vi "Async Serial Engine.vi"(8 "error in (no error)":errorcluster, 10 "Engine Name":string, 11 "Varient Data":variant) -> (0 "error out":errorcluster)   [LabVIEW 2024]
doc: "All Rights Reserved © 2023 SyncSols"
uses:
  Controls/Async State Machine Cases.ctl
  Controls/Async Serial Configuration Cluster.ctl
  Main Engine/Controls/Main Engine JSON Command State.ctl
  Controls/Async Serial Command Q Cluster.ctl
  Main Engine/Controls/Main Engine Engine No.Options.ctl
  TCP Engine/Controls/TCP Engine Serial Interupt Cluster.ctl
  TCP Engine/TCP Engine.lvlib
  Controls/Async Message Info Cluster.ctl
  Controls/Async Frame Info Cluster.ctl
  Main Engine/Controls/Main Engine Q Option.ctl
  Controls/Async Sensor Type.ctl
  <vilib>/Modbus/master/Modbus Master.lvclass
  Controls/Async Serial State Machine Data Cluster.ctl
panel:
  in  "Data Cluster":T1={"Array"=[], "Boolean"=FALSE, "Varient Data"=variant(string ""), "Stop Notification"=refnum, "Start Notification"=refnum, "Command Q"=refnum, "Main Engine Response Q"=refnum, "TCP Engine Response Q"=refnum, "Engine Name"="", "Log File Refnum"=refnum, "Async serial Configuration Cluster"={"Port"="", "Minor Frame Freq"=0, "Minor Frame Count"=0, "Frame Info"=[], "Sensor Type"=0, "OIM Address"=0}, "VISA resource name"="", "Y"=[], "Rate"=0, "Dynamic Data?"=FALSE, "DyData Not Received"=FALSE, "Interupt Q"=refnum, "Modbus"=refnum} {"Async serial Configuration Cluster"."Minor Frame Count" min=5 max=8 step=1}
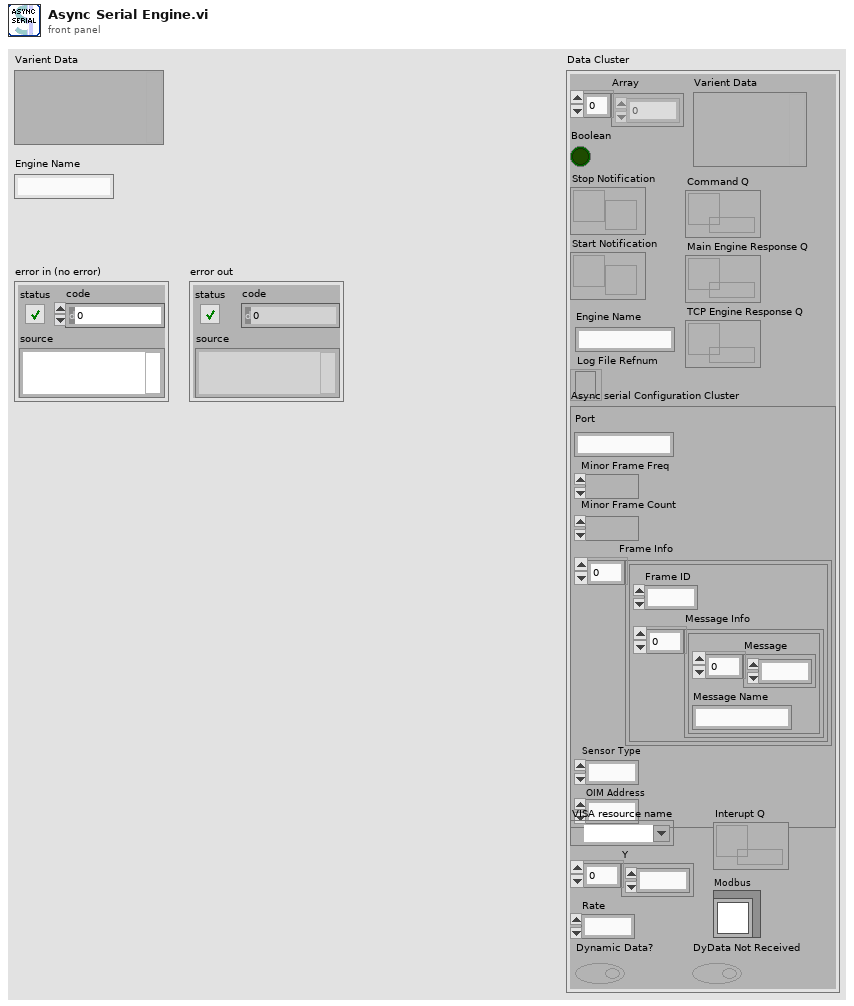
[diagram p1: front panel]
types:
  T1 = typedef "Async Serial State Machine Data Cluster.ctl" = cluster{"Array":dbl[], "Boolean":bool, "Varient Data":variant, "Stop Notification":refnum<notifier>, "Start Notification":refnum<notifier>, "Command Q":refnum<queue>, "Main Engine Response Q":refnum<queue>, "TCP Engine Response Q":refnum<queue>, "Engine Name":string, "Log File Refnum":refnum<file>, "Async serial Configuration Cluster":T2, "VISA resource name":refnum<visa-resource-name>, "Y":dbl[], "Rate":i32, "Dynamic Data?":bool, "DyData Not Received":bool, "Interupt Q":refnum<queue>, "Modbus":refnum<class "Modbus Master.lvclass">}
  T2 = typedef "Async Serial Configuration Cluster.ctl" = cluster{"Port":string, "Minor Frame Freq":u16, "Minor Frame Count":u16, "Frame Info":T3[], "Sensor Type":u16, "OIM Address":u16}
  T3 = typedef "Async Frame Info Cluster.ctl" = cluster{"Frame ID":u16, "Message Info":T4[]}
  T4 = typedef "Async Message Info Cluster.ctl" = cluster{"Message":u8[], "Message Name":string}
  T5 = typedef "Async State Machine Cases.ctl" = enum16{">Poll", ".........State Machine.........", ">Init", ">Error", ">Exit", "..........Async Serial..........", ">JSON to LVData", ">Gen Dyn Data", ">Configure", ">Get Command", ">Write Data"}
  T6 = typedef "Main Engine Q Option.ctl" = enum16{"Init", "Get"}
  T7 = typedef "TCP Engine.lvlib/TCP Engine Serial Interupt Cluster.ctl" = cluster{"Stop":bool, "JSON Variant":variant}
  T8 = typedef "Async Serial Command Q Cluster.ctl" = cluster{"Async serial Configuration Cluster":T2, "Command State":T9}
  T9 = typedef "Main Engine JSON Command State.ctl" = enum16{"Configure", "Start", "Exit"}
  T10 = typedef "Async Sensor Type.ctl" = enum16{"Camera", "INS", "Pri BMS", "Aux BMS", "Depth Sensor", "Altimeter", "OIM", "Thruster", "Acoustic Modem", "LED"}
  T11 = typedef "Main Engine Engine No.Options.ctl" = enum16{"Init", "Update", "Response", "Get"}
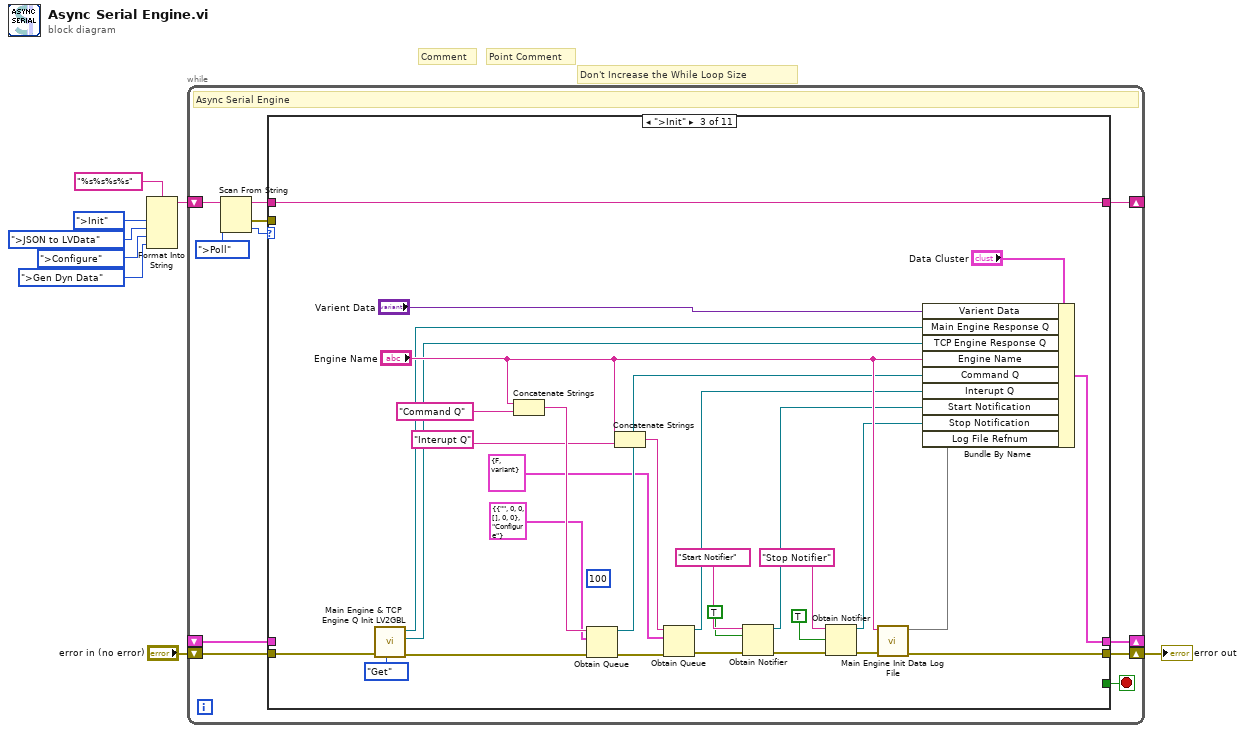
[diagram p0: block diagram]
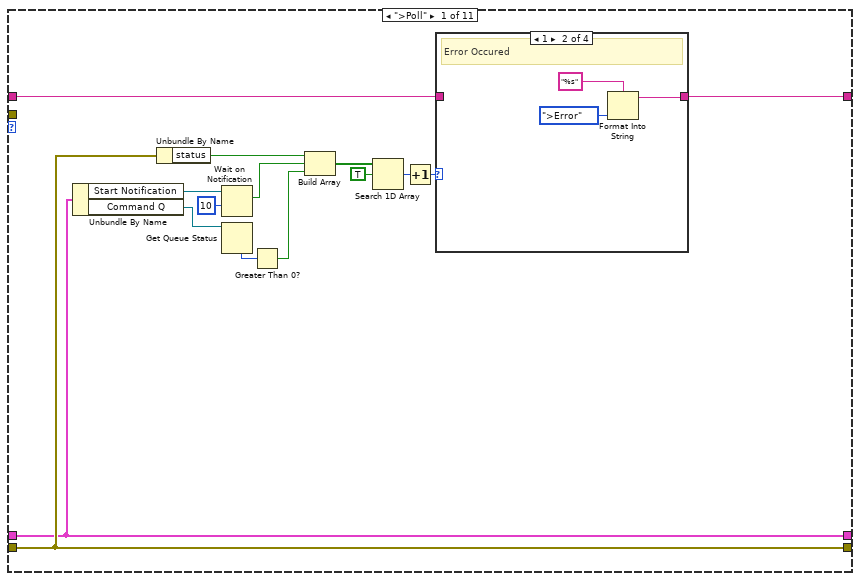
[diagram p2: hidden frame]
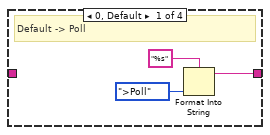
[diagram p3: hidden frame]
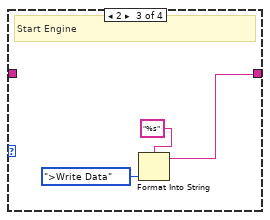
[diagram p4: hidden frame]
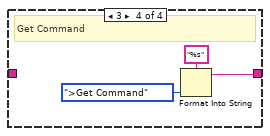
[diagram p5: hidden frame]
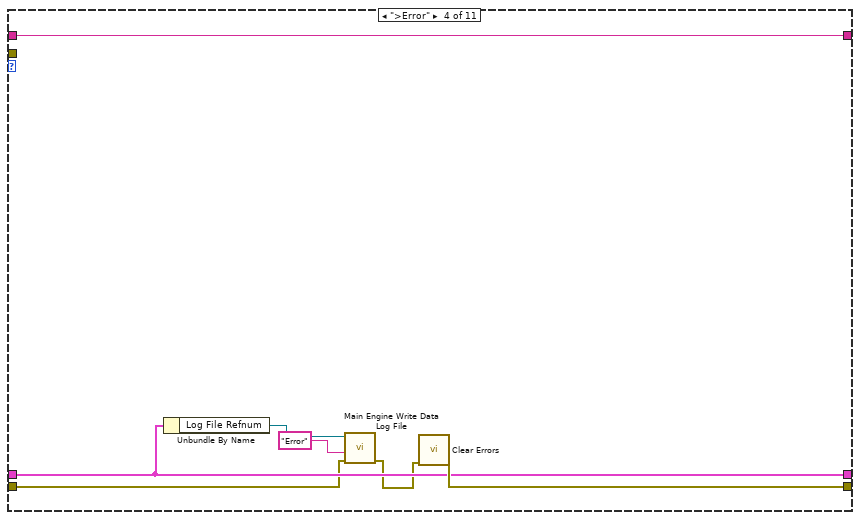
[diagram p7: hidden frame]
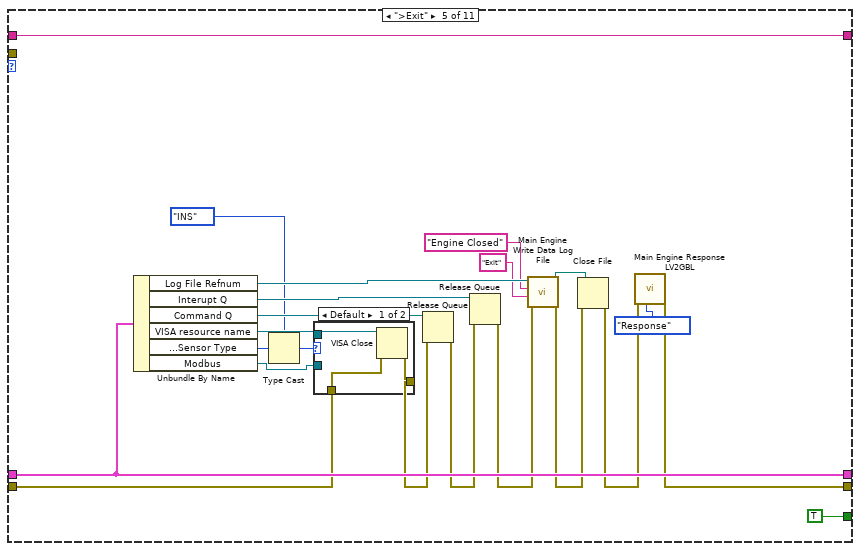
[diagram p8: hidden frame]
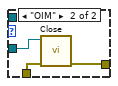
[diagram p9: hidden frame]
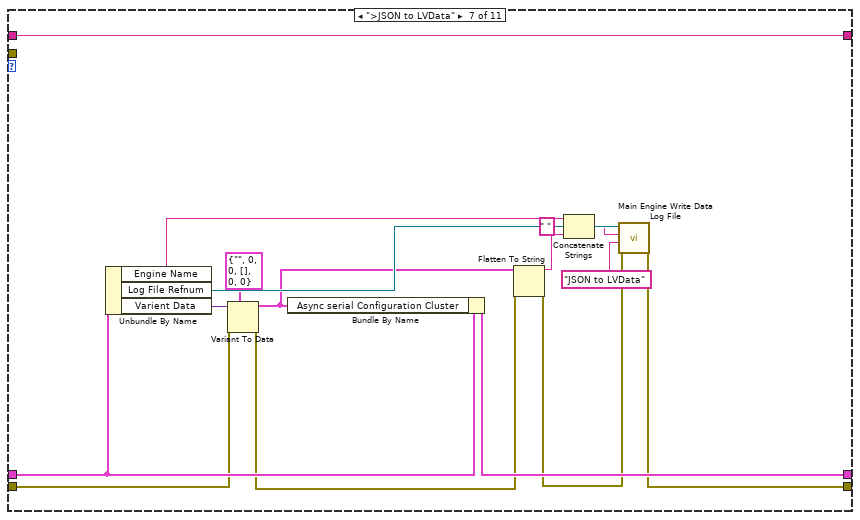
[diagram p11: hidden frame]
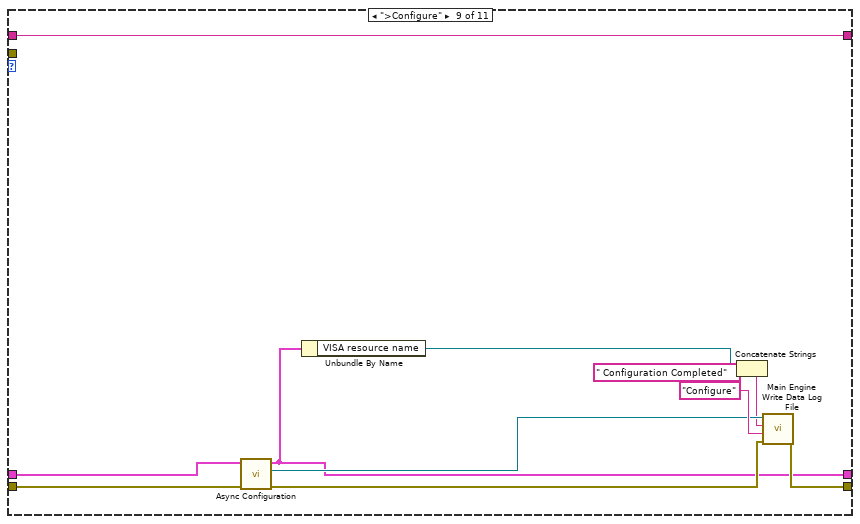
[diagram p13: hidden frame]
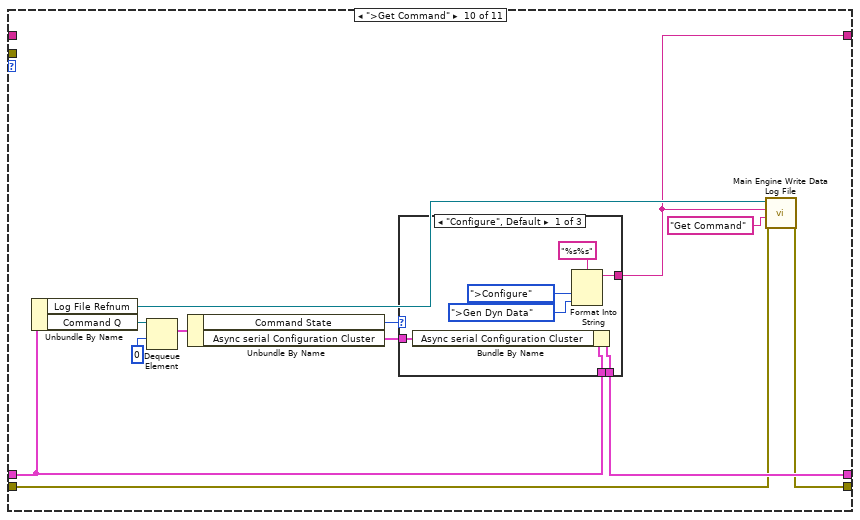
[diagram p14: hidden frame]
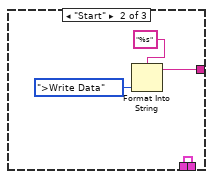
[diagram p15: hidden frame]
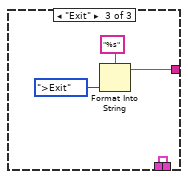
[diagram p16: hidden frame]
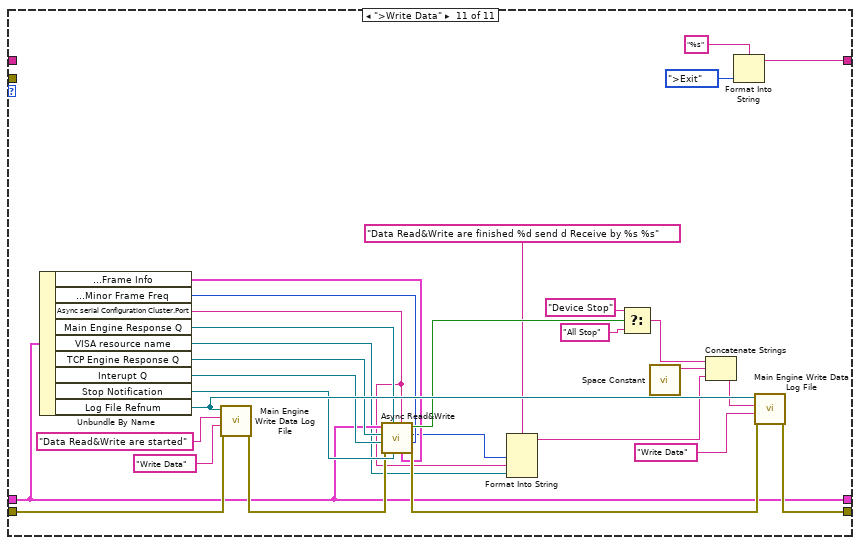
[diagram p17: hidden frame]
diagram:
  # "Don't Increase the While Loop Size"
  # "Point Comment"
  # "Comment"
  n1 = Format Into String(format string="%s%s%s%s", Async_State_Machine_Cases.">Init" ("SM Cases Options"), Async_State_Machine_Cases.">JSON to LVData" ("input 2"), Async_State_Machine_Cases.">Configure" ("input 3"), Async_State_Machine_Cases.">Gen Dyn Data" ("input 3")) -> (resulting string=w7:string)  [unwired: 2 in, 1 out]
  n2 = while {
    shift-right: [w14] -> _
    shift-left: w7 -> [w19]
    shift-right: [w12] -> w4
    shift-left: "error in (no error)" -> [w13]
    shift-right: [w10] -> _
    shift-left: _ -> [w9]
    stop <- w11 stop-if-true
    # "Async Serial Engine"
    n3 = Scan From String(input string=w19, default 1=Async_State_Machine_Cases.">Poll" ("SM Cases Options")) -> (remaining string=w15:string, error out=w17:errorcluster, output 1=w16:T5)  [unwired: 3 in, 1 out]
    n4 = case shown="\">Init\"" w16 {
      tunnel: w17 -> [_ _ _ _ _ _ _ _ _ _ _]
      tunnel: w15 -> [w34 w49 w79 w86 w108 w117 w133 w136 w142 _ _]
      tunnel: [w33 w49 w79 w86 w108 w117 w133 w136 w142 w151 w180] -> w14
      tunnel: w13 -> [w32 w48 w53 w81 w91 w116 w123 w135 w146 w148 w198]
      tunnel: [w32 w48 w65 w85 w95 w116 w128 w135 w144 w149 w203] -> w12
      tunnel: [_ _ _ _ TRUE _ _ _ _ _ _] -> w11
      tunnel: [w26 w47 w63 w82 w106 w115 w130 w134 w139 w154 w178] -> w10
      tunnel: w9 -> [w26 w47 _ w82 w106 w115 w132 w134 w147 w153 w178]
      frame ">Poll" {
        n5 = Unbundle By Name(w26) -> ("Start Notification"=w25:refnum<notifier>, "Command Q"=w24:refnum<queue>)
        n6 = Unbundle By Name(w32) -> ("status"=w31:bool)
        n7 = Wait on Notification(notifier=w25, timeout in ms (-1)=10) -> (notification=w23:bool)  [unwired: 2 in, 3 out]
        n8 = Get Queue Status(queue=w24) -> (# elements in queue=w21:i32)  [unwired: 2 in, 7 out]
        n9 = Greater Than 0?(x=w21) -> (x > 0?=w20:bool)
        n10 = Build Array(w31, w23, w20) -> (w30:bool[])
        n11 = Search 1D Array(1D array=w30, element=TRUE) -> (index of element=w28:i32)  [unwired: 1 in]
        n12 = Increment(x=w28) -> (x+1=w27:i32)
        n13 = case shown="1" w27 {
          tunnel: w34 -> [_ _ _ _]
          tunnel: [w35 w38 w43 w44] -> w33
          frame 0, Default {
            # "Default -> Poll"
            n14 = Format Into String(format string="%s", Async_State_Machine_Cases.">Poll" ("SM Cases Options")) -> (resulting string=w35:string)  [unwired: 2 in, 1 out]
          }
          frame 1 {
            # "Error Occured"
            n15 = Format Into String(format string="%s", Async_State_Machine_Cases.">Error" ("SM Cases Options")) -> (resulting string=w38:string)  [unwired: 2 in, 1 out]
          }
          frame 2 {
            # "Start Engine"
            n16 = Format Into String(format string="%s", Async_State_Machine_Cases.">Write Data" ("SM Cases Options")) -> (resulting string=w43:string)  [unwired: 2 in, 1 out]
          }
          frame 3 {
            # "Get Command"
            n17 = Format Into String(format string="%s", Async_State_Machine_Cases.">Get Command" ("SM Cases Options")) -> (resulting string=w44:string)  [unwired: 2 in, 1 out]
          }
        }
      }
      frame ".........State Machine........." {
      }
      frame ">Init" {
        (unwired) 100 ("max queue size (-1, unlimited)")
        n18 = call "Main Engine & TCP Engine Q Init LV2GBL.vi"("Q Option"=Main_Engine_Q_Option."Get", "error in"=w53) -> ("error out"=w54:errorcluster, "TCP Enigine Tx-Q"=w51:refnum<queue>, "Main Engine Tx-Q"=w52:refnum<queue>)  [unwired: 7 in]
        n19 = Concatenate Strings("Engine Name", "Command Q" ("name (unnamed)")) -> (w69:string)
        n20 = Obtain Queue(name (unnamed)=w69, element data type=T8 {"Async serial Configuration Cluster"={"Port"="", "Minor Frame Freq"=0, "Minor Frame Count"=0, "Frame Info"=[], "Sensor Type"=0, "OIM Address"=0}, "Command State"=enum."Configure"} ("Async Serial Command Q Cluster"), error in (no error)=w54) -> (queue out=w60:refnum<queue>, error out=w77:errorcluster)  [unwired: 2 in, 1 out]
        n21 = Concatenate Strings("Engine Name", "Interupt Q" ("name (unnamed)")) -> (w67:string)
        n22 = Obtain Queue(name (unnamed)=w67, element data type=T7 {"Stop"=FALSE, "JSON Variant"=variant} ("Serial Interupt Cluster"), error in (no error)=w77) -> (queue out=w55:refnum<queue>, error out=w76:errorcluster)  [unwired: 2 in, 1 out]
        n23 = Obtain Notifier(name (unnamed)="Start Notifier", notification data type=TRUE, error in (no error)=w76) -> (notifier out=w59:refnum<notifier>, error out=w75:errorcluster)  [unwired: 1 in, 1 out]
        n24 = Obtain Notifier(name (unnamed)="Stop Notifier", notification data type=TRUE, error in (no error)=w75) -> (notifier out=w58:refnum<notifier>, error out=w66:errorcluster)  [unwired: 1 in, 1 out]
        n25 = call "Main Engine Init Data Log File.vi"("error in"=w66, "Engine Name"="Engine Name") -> ("error out"=w65:errorcluster, 3:w57)  [unwired: 7 in, 1 out]
        n26 = Bundle By Name(cluster="Data Cluster", "Varient Data"="Varient Data", "Main Engine Response Q"=w52, "TCP Engine Response Q"=w51, "Engine Name"="Engine Name", "Command Q"=w60, "Interupt Q"=w55, "Start Notification"=w59, "Stop Notification"=w58, "Log File Refnum"=w57) -> (w63:T1)
      }
      frame ">Error" {
        n27 = Unbundle By Name(w82) -> ("Log File Refnum"=w84:refnum<file>)
        n28 = call "Main Engine Write Data Log File.vi"("error in"=w81, "State"="Error" ("Input Data"), "Log file path In"=w84) -> ("error out"=w80:errorcluster)  [unwired: 7 in, 1 out]
        n29 = call <vilib>:"Clear Errors.vi"("error in (no error)"=w80) -> ("error out"=w85:errorcluster)  [unwired: 5 in, 1 out]
      }
      frame ">Exit" {
        n30 = Unbundle By Name(w106) -> ("Log File Refnum"=w102:refnum<file>, "Interupt Q"=w93:refnum<queue>, "Command Q"=w103:refnum<queue>, "VISA resource name"=w92:refnum<visa-resource-name>, "Async serial Configuration Cluster.Sensor Type"=w90:u16, "Modbus"=w87:refnum<class "Modbus Master.lvclass">)
        n31 = Type Cast(type=Async_Sensor_Type."INS" ("Sensor Type"), x=w90) -> (*(type *) &x=w89:T10)
        n32 = case shown="Default" w89 {
          tunnel: [w111 w113] -> w105
          tunnel: w92 -> [w110 _]
          tunnel: w91 -> [w109 w114]
          tunnel: w87 -> [_ w112]
          frame Default {
            n33 = VISA Close(VISA resource name=w110, error in (no error)=w109) -> (error out=w111:errorcluster)
          }
          frame "OIM" {
            n34 = call-dynamic "Close.vi"("error in (no error)"=w114, "Modbus master in"=w112) -> ("error out"=w113:errorcluster)  [unwired: 9 in]
          }
        }
        n35 = Release Queue(queue=w103, error in (no error)=w105) -> (error out=w104:errorcluster)  [unwired: 1 in, 2 out]
        n36 = Release Queue(queue=w93, error in (no error)=w104) -> (error out=w101:errorcluster)  [unwired: 1 in, 2 out]
        n37 = call "Main Engine Write Data Log File.vi"("error in"=w101, "State"="Exit", "Input Data"="Engine Closed", "Log file path In"=w102) -> ("error out"=w100:errorcluster, "Log File Path Out"=w99:path)  [unwired: 6 in]
        n38 = Close File(refnum=w99, error in=w100) -> (error out=w96:errorcluster)  [unwired: 1 out]
        n39 = call "Main Engine Response LV2GBL.vi"("Options"=Main_Engine_Engine_No.Options."Response", "error in"=w96) -> ("error out"=w95:errorcluster)  [unwired: 7 in, 2 out]
      }
      frame "..........Async Serial.........." {
      }
      frame ">JSON to LVData" {
        n40 = Unbundle By Name(w132) -> ("Engine Name"=w119:string, "Log File Refnum"=w129:refnum<file>, "Varient Data"=w131:variant)
        n41 = Variant To Data(error in=w123, type=T2 {"Port"="", "Minor Frame Freq"=0, "Minor Frame Count"=0, "Frame Info"=[], "Sensor Type"=0, "OIM Address"=0} ("Async serial Configuration Cluster"), Variant=w131) -> (data=w121:T2, error out=w122:errorcluster)
        n42 = Bundle By Name(cluster=w132, "Async serial Configuration Cluster"=w121) -> (w130:T1)
        n43 = Flatten To String(anything=w121, error in (no error)=w122) -> (data string=w125:string, error out=w126:errorcluster)  [unwired: 2 in, 1 out]
        n44 = Concatenate Strings(w119, " " ("string"), w125) -> (w120:string)
        n45 = call "Main Engine Write Data Log File.vi"("error in"=w126, "State"="JSON to LVData", "Input Data"=w120, "Log file path In"=w129) -> ("error out"=w128:errorcluster)  [unwired: 6 in, 1 out]
      }
      frame ">Gen Dyn Data" {
      }
      frame ">Configure" {
        n46 = call "Async Configuration.vi"("error in"=w146, "Data Cluster in"=w147) -> ("error out"=w143:errorcluster, "File out"=w140:refnum<file>, "Data Cluster out"=w139:T1)  [unwired: 7 in]
        n47 = Unbundle By Name(w139) -> ("VISA resource name"=w137:refnum<visa-resource-name>)
        n48 = Concatenate Strings(w137, " Configuration Completed" ("Input Data")) -> (w138:string)
        n49 = call "Main Engine Write Data Log File.vi"("error in"=w143, "State"="Configure", "Input Data"=w138, "Log file path In"=w140) -> ("error out"=w144:errorcluster)  [unwired: 6 in, 1 out]
      }
      frame ">Get Command" {
        n50 = Unbundle By Name(w153) -> ("Log File Refnum"=w152:refnum<file>, "Command Q"=w159:refnum<queue>)
        n51 = Dequeue Element(queue=w159, timeout in ms (-1)=0) -> (element=w157:T8)  [unwired: 1 in, 3 out]
        n52 = Unbundle By Name(w157) -> ("Command State"=w156:T9, "Async serial Configuration Cluster"=w155:T2)
        n53 = case shown="\"Configure\", Default" w156 {
          tunnel: w153 -> [w166 w170 w174]
          tunnel: w155 -> [w165 _ _]
          tunnel: [w164 w170 w174] -> w154
          tunnel: [w161 w169 w171] -> w151
          frame "Configure", Default {
            n54 = Bundle By Name(cluster=w166, "Async serial Configuration Cluster"=w165) -> (w164:T1)
            n55 = Format Into String(format string="%s%s", Async_State_Machine_Cases.">Configure" ("SM Cases Options"), Async_State_Machine_Cases.">Gen Dyn Data" ("SM Cases Options")) -> (resulting string=w161:string)  [unwired: 2 in, 1 out]
          }
          frame "Start" {
            n56 = Format Into String(format string="%s", Async_State_Machine_Cases.">Write Data" ("SM Cases Options")) -> (resulting string=w169:string)  [unwired: 2 in, 1 out]
          }
          frame "Exit" {
            n57 = Format Into String(format string="%s", Async_State_Machine_Cases.">Exit" ("SM Cases Options")) -> (resulting string=w171:string)  [unwired: 2 in, 1 out]
          }
        }
        n58 = call "Main Engine Write Data Log File.vi"("error in"=w148, "State"="Get Command", "Input Data"=w151, "Log file path In"=w152) -> ("error out"=w149:errorcluster)  [unwired: 6 in, 1 out]
      }
      frame ">Write Data" {
        n59 = Unbundle By Name(w178) -> ("Async serial Configuration Cluster.Frame Info"=w184:T3[], "Async serial Configuration Cluster.Minor Frame Freq"=w183:u16, "Async serial Configuration Cluster.Port"=w176:string, "Main Engine Response Q"=w192:refnum<queue>, "VISA resource name"=w175:refnum<visa-resource-name>, "TCP Engine Response Q"=w191:refnum<queue>, "Interupt Q"=w190:refnum<queue>, "Stop Notification"=w189:refnum<notifier>, "Log File Refnum"=w199:refnum<file>)
        n60 = call "Main Engine Write Data Log File.vi"("error in"=w198, "State"="Write Data", "Input Data"="Data Read&Write are started", "Log file path In"=w199) -> ("error out"=w179:errorcluster)  [unwired: 6 in, 1 out]
        n61 = call "Async Read&Write.vi"("Minor Frame Freq"=w183, "Frame Info Array"=w184, "Port"=w176, "Stop Notification"=w189, "Main Engine Response Q"=w192, "error in"=w179, "Interupt Q"=w190, "TCP Engine Response Q"=w191, "Data Cluster"=w178) -> ("error out"=w188:errorcluster, "Total # Send"=w177:i32, "Device Stop"=w187:bool)
        n62 = Format Into String(format string="Data Read&Write are finished %d send d Receive by %s %s" ("Input Data"), w177, w176, w175) -> (resulting string=w185:string)  [unwired: 2 in, 1 out]
        n63 = Select(t="Device Stop" ("Input Data"), s=w187, f="All Stop" ("Input Data")) -> (s? t:f=w195:string)
        n64 = call <vilib>:"Space Constant.vi"() -> ("String"=w193:string)
        n65 = Concatenate Strings(w195, w193, w185) -> (w194:string)
        n66 = Format Into String(format string="%s", Async_State_Machine_Cases.">Exit" ("SM Cases Options")) -> (resulting string=w180:string)  [unwired: 2 in, 1 out]
        n67 = call "Main Engine Write Data Log File.vi"("error in"=w188, "State"="Write Data", "Input Data"=w194, "Log file path In"=w199) -> ("error out"=w203:errorcluster)  [unwired: 6 in, 1 out]
      }
    }
  }
  "error out" <- w4
